vi "Scratchpad.vi"() -> ()   [LabVIEW 2022 SP3]
uses:
  open-hw-mon-lv/OpenHW/HW Node.ctl
  open-hw-mon-lv/OpenHW/OpenHW.lvclass
panel:
  in  "Children Names":string[](array[string])
  out "HW by Names":T1
  in  "Children Indices":i32[](array[numeric])=[0, 1, 1, 0]
  out "HW by Indices":T1
  in  "Tree":string(tree)
  out "error out":errorcluster
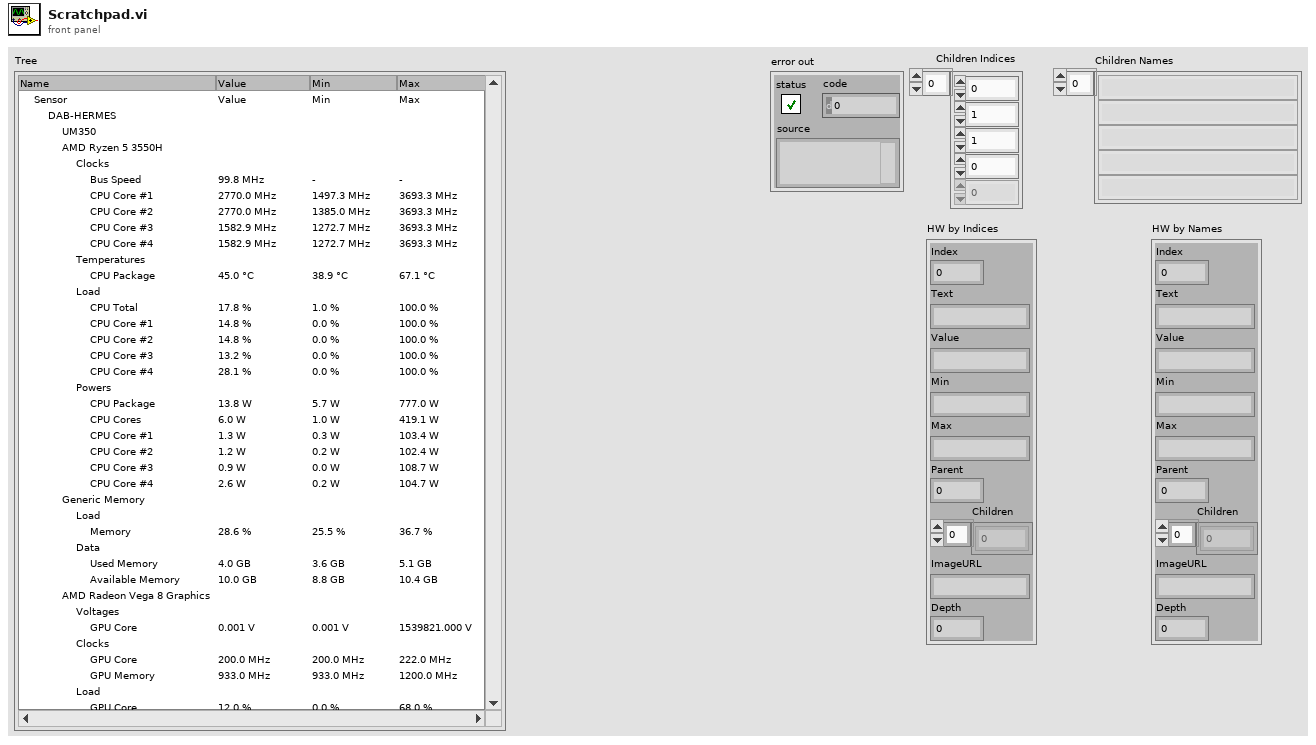
[diagram p1: front panel]
types:
  T1 = typedef "open-hw-mon-lv.lvlib/OpenHW.lvclass/HW Node.ctl" = cluster{"Index":i32, "Text":string, "Value":string, "Min":string, "Max":string, "Parent":i32, "Children":i32[], "ImageURL":string, "Depth":i32}
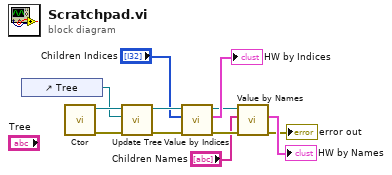
[diagram p0: block diagram]
diagram:
  n1 = control-ref of="Tree"() -> (w11:refnum<vi>)
  n2 = call "Ctor.vi"() -> ("error out"=w10:errorcluster, "OpenHW out"=w12:refnum<class "OpenHW.lvclass">)  [unwired: 10 in]
  n3 = call "Update Tree.vi"("error in (no error)"=w10, "Tree"=w11, "OpenHW in"=w12) -> ("error out"=w8:errorcluster, "OpenHW out"=w9:refnum<class "OpenHW.lvclass">)  [unwired: 7 in]
  n4 = call "Value by Indices.vi"("error in (no error)"=w8, "Children Indices"="Children Indices", "OpenHW in"=w9) -> ("error out"=w4:errorcluster, "HW Node"=→"HW by Indices":T1, "OpenHW out"=w5:refnum<class "OpenHW.lvclass">)  [unwired: 6 in]
  n5 = call "Value by Names.vi"("error in (no error)"=w4, "Children Names"="Children Names", "OpenHW in"=w5) -> ("error out"=→"error out":errorcluster, "HW Node"=→"HW by Names":T1)  [unwired: 6 in, 1 out]
